vi "PathPlanner_PathFinder_ApplyControlSmooth.vi"(10 "Current":T1 {"Y" format="%14.3f"; "X" format="%14.3f"}, 11 "Other":T1 {"Y" format="%14.3f"; "X" format="%14.3f"}) -> (3 "Smoothed":T1 {"Y" format="%14.3f"; "X" format="%14.3f"})   [LabVIEW 2019, in "PathPlanner24.lvlib"]
uses:
  <vilib>/Rock Robotics/WPI/ThirdParty/JAS_Junk/TrajLib/TypeDef/TRANSLATION2D.ctl
  <vilib>/Rock Robotics/WPI/ThirdParty/JAS_Junk/TrajLib/Translation2d_Create.vi
  PathPlanner24.lvlib
  <vilib>/Rock Robotics/WPI/ThirdParty/JAS_Junk/TrajLib/Trajectory_Library.lvlib
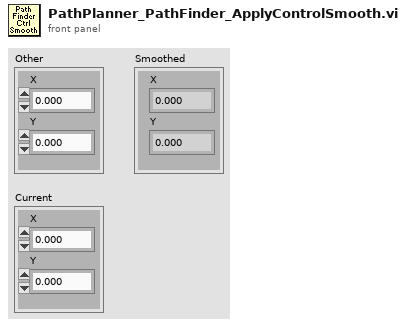
[diagram p1: front panel]
types:
  T1 = typedef "Trajectory_Library.lvlib/TRANSLATION2D.ctl" = cluster{"X":dbl, "Y":dbl}
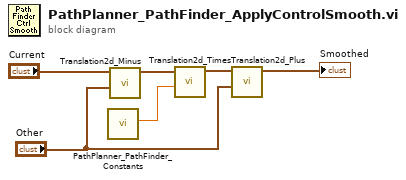
[diagram p0: block diagram]
diagram:
  n1 = call "PathPlanner_PathFinder_Constants.vi"() -> ("SMOOTHING_CONTROL_PCT"=w1:dbl)  [unwired: 9 in, 2 out]
  n2 = call <vilib>:"Translation2d_Minus.vi"("other Translation"="Other", "In Translation"="Current") -> ("Out Translation"=w3:T1)  [unwired: 9 in]
  n3 = call <vilib>:"Translation2d_Times.vi"("Scalar"=w1, "In Translation"=w3) -> ("Out Translation"=w4:T1)  [unwired: 9 in]
  n4 = call <vilib>:"Translation2d_Plus.vi"("other Translation"="Other", "In Translation"=w4) -> ("Out Translation"=→"Smoothed":T1)  [unwired: 9 in]
